vi "Add Text to Today's Page.vi"(5 "Alignment":string="left", 6 "Font Size":string="12", 7 "Color":string="black", 8 "Error In (No Error)":errorcluster, 9 "Your Text Here":string, 10 "Notebook Name":string="My notebook on One Drive", 11 "User Email":string="myemail") -> (0 "error out":errorcluster, 2 "body":string, 3 "headers":string)   [LabVIEW 2019, in "OneNote Library.lvlib"]
uses:
  OneNote Library.lvlib
  Useful OAuth VIs/globals.vi
  <vilib>/httpClient/POSTBuffer.vi
  <vilib>/httpClient/LabVIEWHTTPClient.lvlib
  Useful OAuth VIs/Useful OAuth VIs.lvlib
panel:
  out "Page ID":string
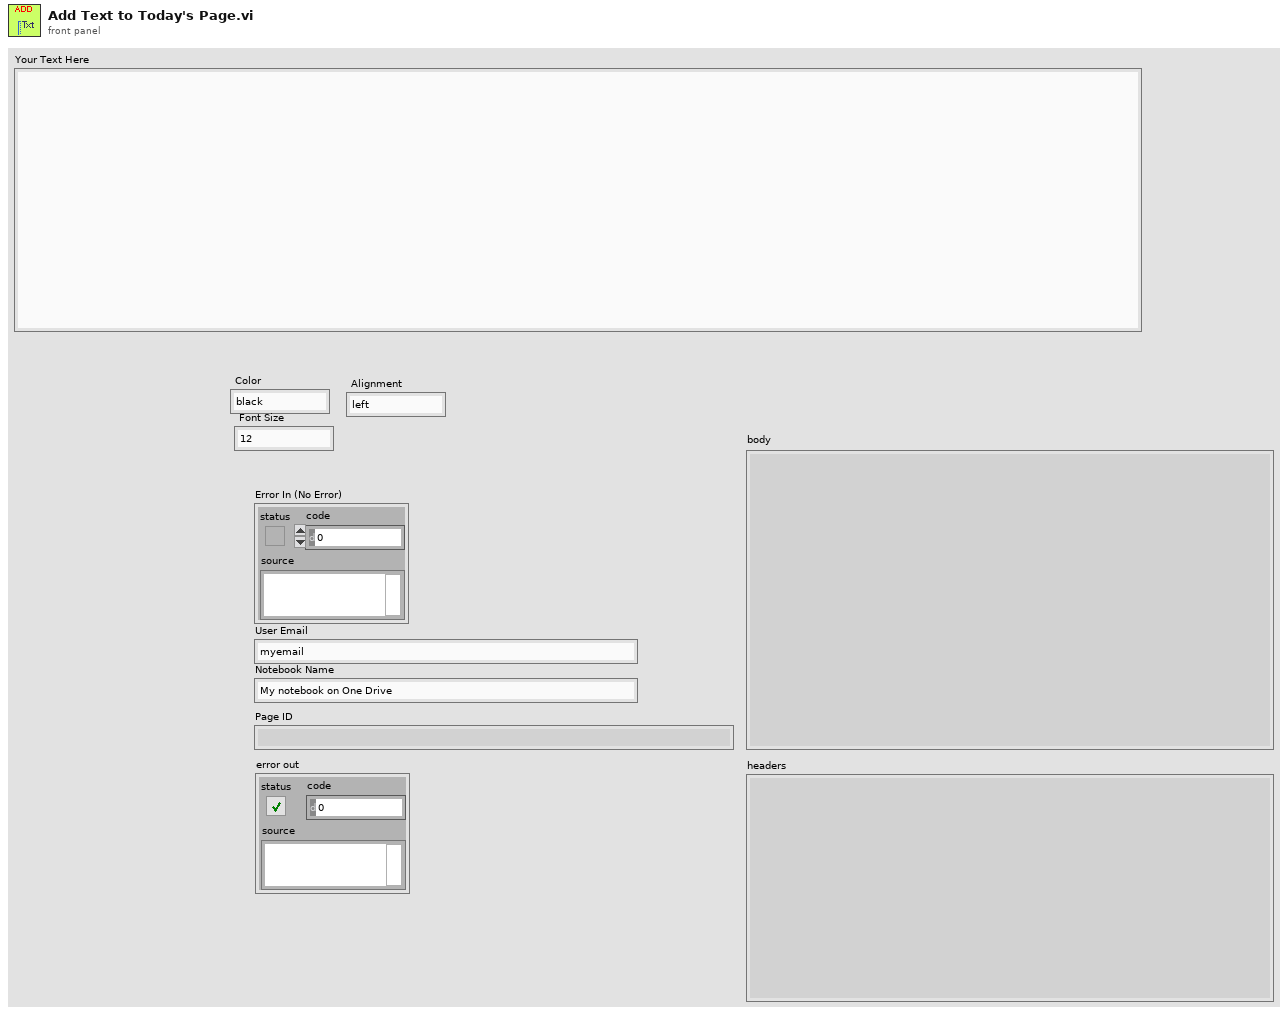
[diagram p1: front panel]
types:
  T1 = typedef "LabVIEWHTTPClient.lvlib/ClientHandle.ctl" = refnum<k1>
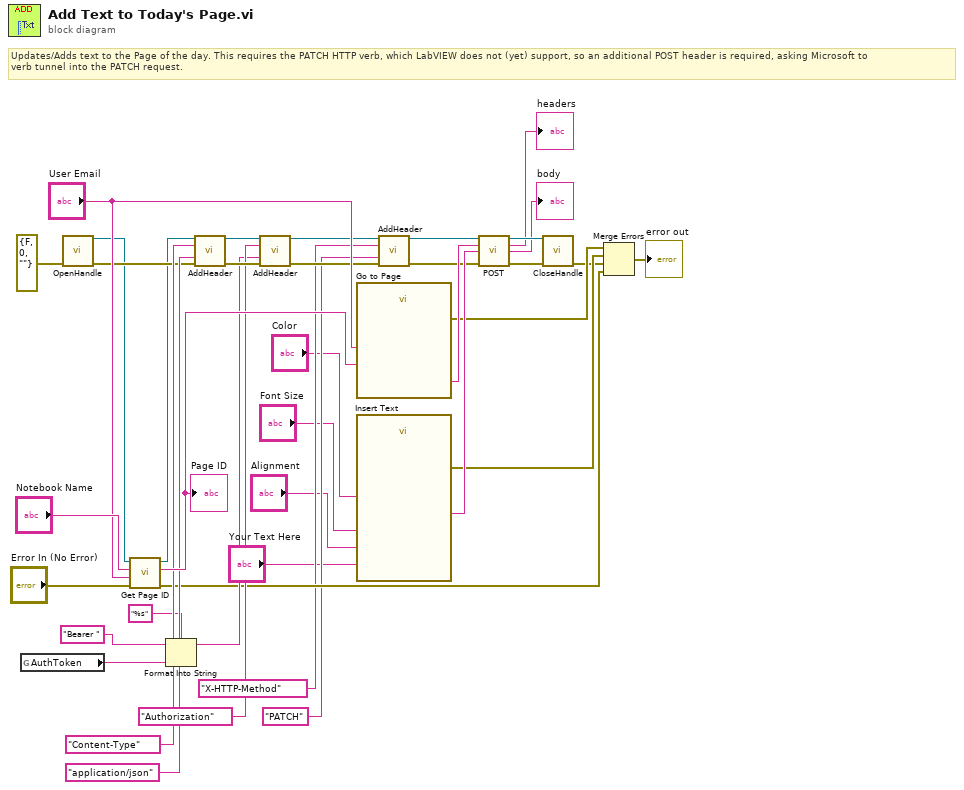
[diagram p0: block diagram]
diagram:
  # "Updates/Adds text to the Page of the day. This requires the PATCH HTTP verb, which LabVIEW does not (yet) support, so an additional POST header is required, asking Microsoft to \nverb tunnel into the PATCH request."
  n1 = global read "globals.vi" "AuthToken"() -> (w25:string)
  n2 = call <vilib>:"OpenHandle.vi"("error in (no error)"=errorcluster {"status"=FALSE, "code"=0, "source"=""}) -> ("client handle out"=w15:T1, "error out"=w30:errorcluster)  [unwired: 13 in]
  n3 = call "Get Page ID.vi"("Error In (No Error)"="Error In (No Error)", "User Email"="User Email", "Notebook Name"="Notebook Name", "client handle"=w15) -> ("error out"=w16:errorcluster, "Page ID"=w35:string, "client handle out"=w14:T1)  [unwired: 5 in]
  "Page ID" <- w35
  n4 = Format Into String(format string="%s", initial string="Bearer ", w25) -> (resulting string=w26:string)  [unwired: 1 in, 1 out]
  n5 = call <vilib>:"AddHeader.vi"("client handle"=w14, "header"="Content-Type", "value"="application/json", "error in (no error)"=w30) -> ("client handle out"=w32:T1, "error out"=w31:errorcluster)  [unwired: 10 in]
  n6 = call <vilib>:"AddHeader.vi"("client handle"=w32, "header"="Authorization", "value"=w26, "error in (no error)"=w31) -> ("client handle out"=w11:T1, "error out"=w10:errorcluster)  [unwired: 10 in]
  n7 = call "Go to Page"("user"="User Email", "Page ID"=w35) -> ("Result"=w24:string, "error out"=w20:errorcluster)  [unwired: 12 in]
  n8 = call "Insert Text"("Your Text Here"="Your Text Here", "Color"="Color", "Font Size"="Font Size", "Alignment"="Alignment") -> ("Result"=w23:string, "error out"=w19:errorcluster)  [unwired: 10 in]
  n9 = call <vilib>:"AddHeader.vi"("client handle"=w11, "header"="X-HTTP-Method", "value"="PATCH", "error in (no error)"=w10) -> ("client handle out"=w9:T1, "error out"=w8:errorcluster)  [unwired: 10 in]
  n10 = call-poly <vilib>:"POST.vi"("client handle"=w9, "url"=w24, "buffer"=w23, "error in (no error)"=w8) -> ("client handle out"=w22:T1, "headers"=→"headers":string, "body"=→"body":string, "error out"=w21:errorcluster)  [unwired: 8 in]
  n11 = call <vilib>:"CloseHandle.vi"("client handle"=w22, "error in (no error)"=w21) -> ("error out"=w18:errorcluster)  [unwired: 13 in]
  n12 = Merge Errors(w20, w19, w18, w16) -> (→"error out":errorcluster)
